vi "Color Sensor V3 Get Raw Color.vi"(8 "error in (no error)":errorcluster, 11 "ColorSensorDevRef":T2={"I2CDevRef"={"DevStatus"={"status"=FALSE, "code"=0, "source"=""}, "Device Address"=0, "Handle"=0, "I2C Bus"=enum."Invalid"}} {"I2CDevRef"."Device Address" format="%.0x"}) -> (0 "error out":errorcluster, 2 "Raw Color":T1, 3 "ColorSensorDevRef out":T2={"I2CDevRef"={"DevStatus"={"status"=FALSE, "code"=0, "source"=""}, "Device Address"=0, "Handle"=0, "I2C Bus"=enum."Invalid"}} {"I2CDevRef"."Device Address" format="%.0x"})   [LabVIEW 2019]
uses:
  TypeDef/Color Sensor V3 DevRef.ctl
  <vilib>/Rock Robotics/WPI/I2C/WPI_I2CDevRef.ctl
  <vilib>/Rock Robotics/SystemInterfaces/i2clib/i2c_bus.ctl
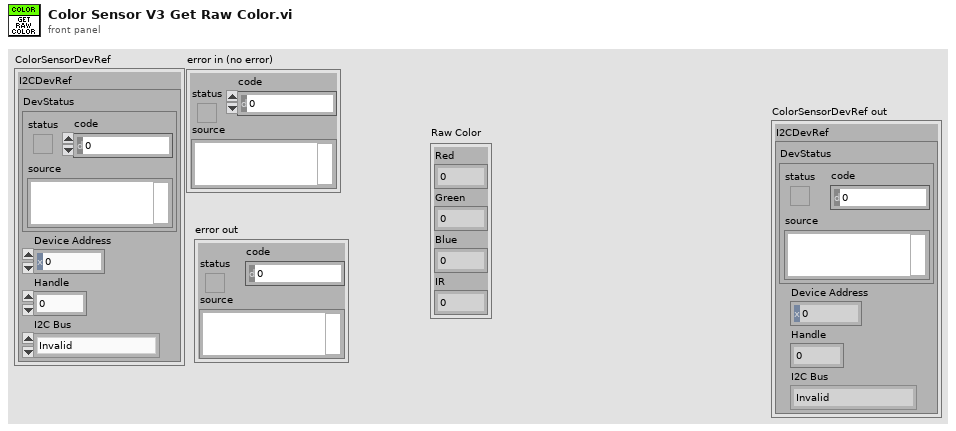
[diagram p1: front panel]
types:
  T1 = cluster{"Red":u32, "Green":u32, "Blue":u32, "IR":u32}
  T2 = typedef "Color Sensor V3 DevRef.ctl" = cluster{"I2CDevRef":T3}
  T3 = typedef "WPI_I2CDevRef.ctl" = cluster{"DevStatus":errorcluster, "Device Address":u8, "Handle":i32, "I2C Bus":T4}
  T4 = typedef "i2c_bus.ctl" = enum16{"I2C On-Board", "I2C MXP", "Invalid"}
  T5 = cluster{"Result":u32, "Result":u32, "Result":u32, "Result":u32}
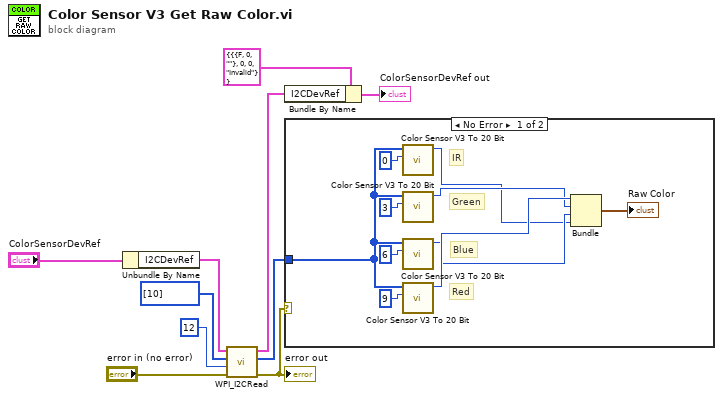
[diagram p0: block diagram]
diagram:
  n1 = Unbundle By Name("ColorSensorDevRef") -> ("I2CDevRef"=w7:T3)
  n2 = call <vilib>:"WPI_I2CRead.vi"("error in (no error)"="error in (no error)", "I2CBytesToRead"=u8 12, "I2CRegister"=u8[] [10], "I2CDevRef"=w7) -> ("error out"=w5:errorcluster, "Data Out"=w4:u8[], "I2CDevRef"=w2:T3)  [unwired: 5 in]
  "error out" <- w5
  n3 = Bundle By Name(cluster=T2 {"I2CDevRef"={"DevStatus"={"status"=FALSE, "code"=0, "source"=""}, "Device Address"=0, "Handle"=0, "I2C Bus"=enum."Invalid"}} ("ColorSensorDevRef 2"), "I2CDevRef"=w2) -> (→"ColorSensorDevRef out":T2)
  n4 = case shown="No Error" w5 {
    tunnel: w4 -> [w20 _]
    frame No Error {
      # "Red"
      # "Blue"
      # "Green"
      # "IR"
      n5 = call "Color Sensor V3 To 20 Bit.vi"("index (0)"=0 ("index"), "array"=w20) -> ("Result"=w11:u32)  [unwired: 9 in]
      n6 = call "Color Sensor V3 To 20 Bit.vi"("index (0)"=3 ("index"), "array"=w20) -> ("Result"=w13:u32)  [unwired: 9 in]
      n7 = call "Color Sensor V3 To 20 Bit.vi"("index (0)"=6 ("index"), "array"=w20) -> ("Result"=w12:u32)  [unwired: 9 in]
      n8 = call "Color Sensor V3 To 20 Bit.vi"("index (0)"=9 ("index"), "array"=w20) -> ("Result"=w15:u32)  [unwired: 9 in]
      n9 = Bundle("Result"=w15, "Result"=w13, "Result"=w12, "Result"=w11) -> (→"Raw Color":T5)  [unwired: 1 in]
    }
    frame Error {
    }
  }
